vi "BPCS-Malicious-DE.vi"() -> ()   [LabVIEW 2017]
uses:
  <vilib>/Platform/TimedLoop/XDataNode/timing_clust.ctl
  <vilib>/Platform/TimedLoop/XDataNode/nitl_modes.ctl
  <vilib>/Platform/TimedLoop/XDataNode/wakeup.ctl
  <vilib>/addons/control/pid/pid.llb/PID Advanced (DBL).vi
  <vilib>/Platform/TimedLoop/XDataNode/XDataNode.xnode
  <vilib>/Platform/TimedLoop/XDataNode/XDNodeRunTimeDep.lvlib
  <vilib>/addons/control/pid/NI_PID_pid.lvlib
panel:
  in  "stop":bool
  out "data out":string
  in  "Stop":bool
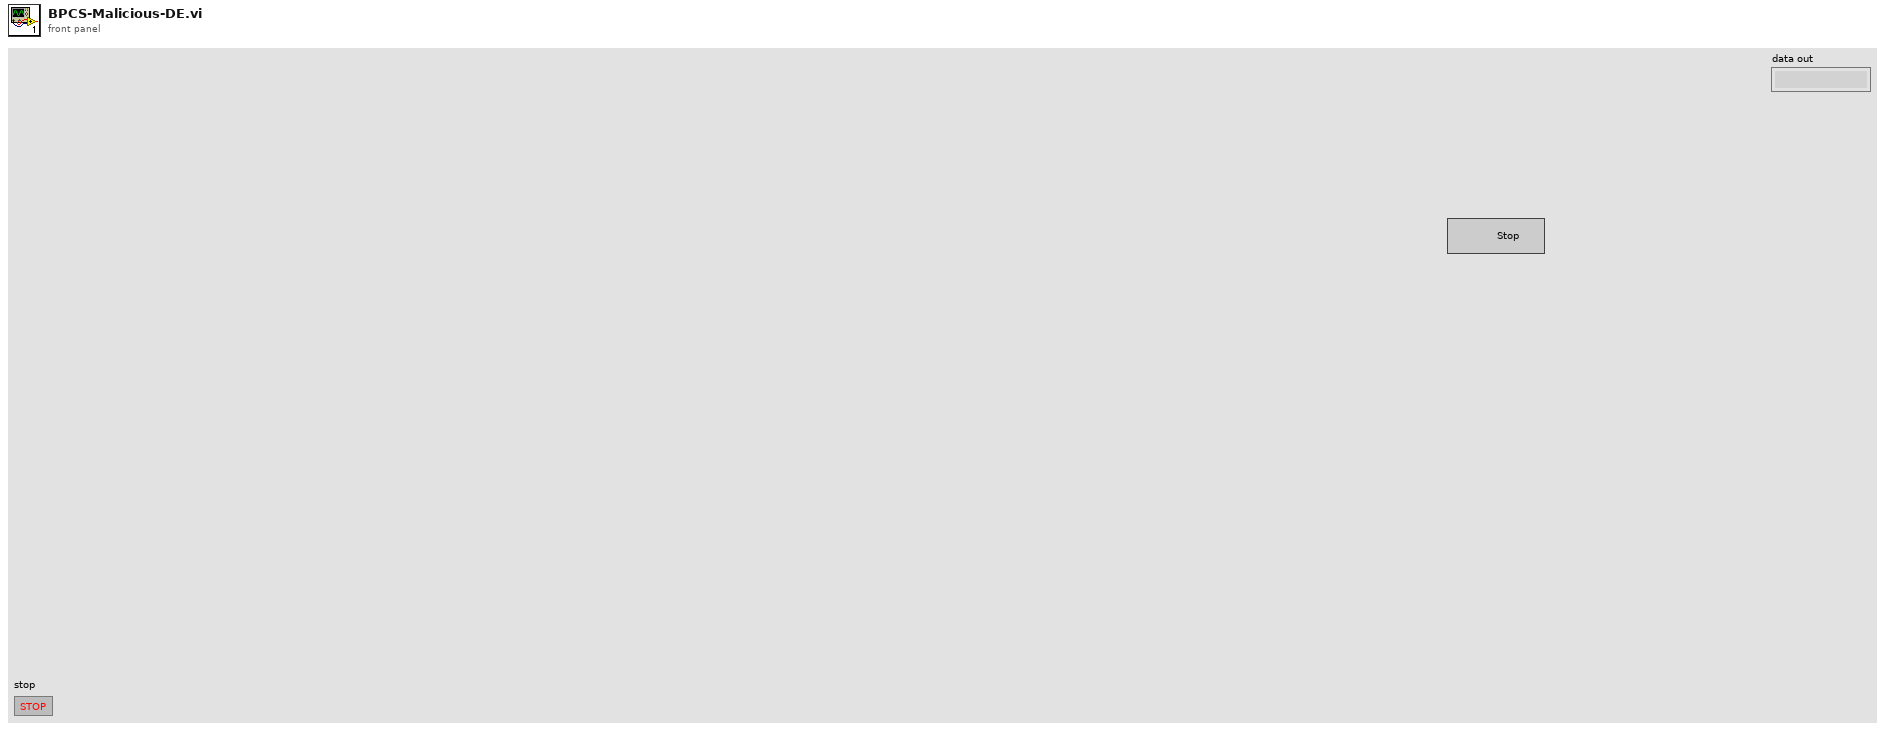
[diagram p1: front panel]
types:
  T1 = typedef "XDNodeRunTimeDep.lvlib/timing_clust.ctl" = cluster{"Expected End [f-1]":u64, "Actual End [f-1]":u64, "Finished Late? [f-1]":bool, "Expected End [i-1]":u64, "Actual End [i-1]":u64, "Finished Late? [i-1]":bool, "Expected Start [i]":u64, "Actual Start [i]":u64, "Expected Start [f]":u64, "Actual Start [f]":u64, "Source Name":string, "Structure Name":string, "Period":i64, "Deadline":i64, "Offset":i64, "Start":i64, "Priority":i32, "Timeout":i32, "Mode":T2, "Wakeup Reason":T3, "Error":errorcluster, "Source Type":string, "Secondary Source Type":string, "Global End Time":u64, "Global Start Time":u64, "Frame Duration":u64, "Iteration Duration":u64, "Assigned CPU":i32, "I/O Scan Engine Mode":u32}
  T2 = typedef "XDNodeRunTimeDep.lvlib/nitl_modes.ctl" = enum32{"No Change", "Process missed periods, maintain original phase", "Discard missed periods, maintain original phase", "Process missed periods, ignore original phase", "Discard missed periods, ignore original phase"}
  T3 = typedef "XDNodeRunTimeDep.lvlib/wakeup.ctl" = enum32{"Normal", "Aborted", "Asynchronous wakeup", "Timing source error", "Timed loop error", "Timeout"}
  T4 = cluster{"Array of Double[0]":dbl, "Array of Double[1]":dbl, "Array of Double[2]":dbl}
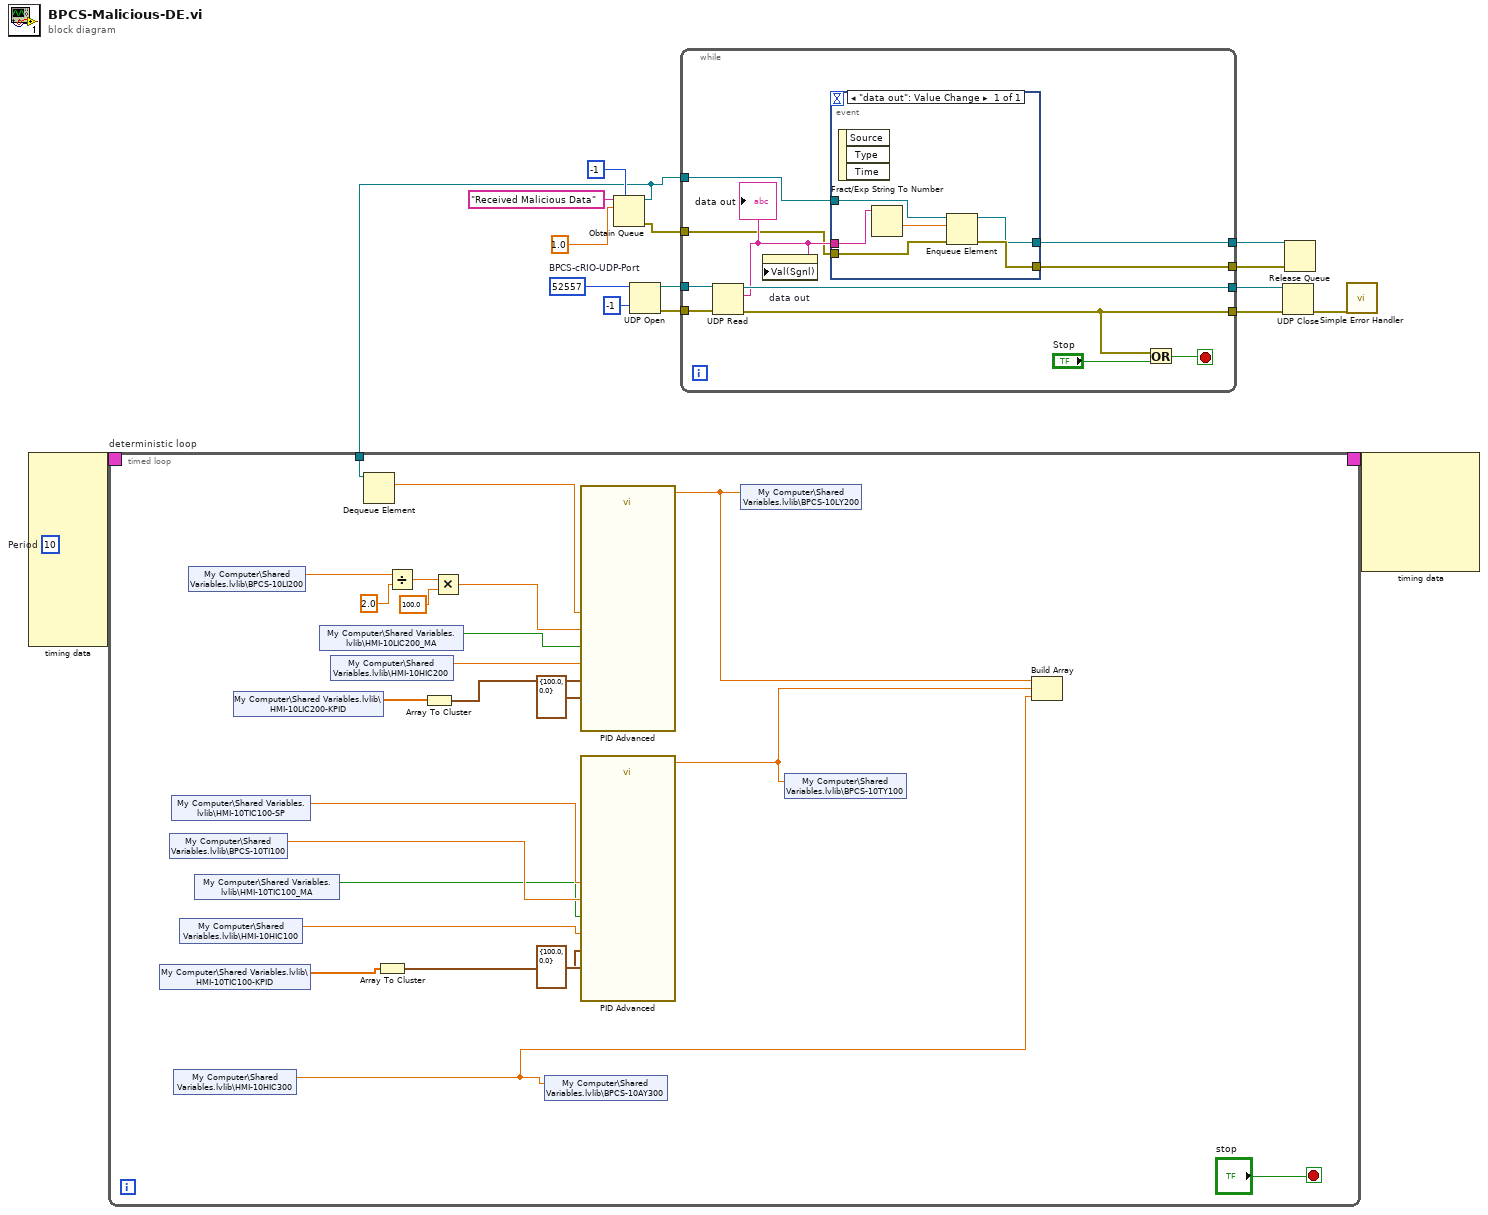
[diagram p0: block diagram]
diagram:
  w2 = i64 10  # Period
  w17 = u16 52557  # BPCS-cRIO-UDP-Port
  n1 = node-c288 ("Input Node")(w2) -> (w4:T1)  [unwired: 9 in]
  n2 = Obtain Queue(max queue size (-1, unlimited)=-1, name (unnamed)="Received Malicious Data", element data type=1.0) -> (queue out=w1:refnum<queue>, error out=w5:errorcluster)  [unwired: 2 in, 1 out]
  n3 = timed-loop "deterministic loop" {
    timing: w4 -> [_]
    timing-out: [_] -> w3
    tunnel: w1 -> [w19]
    stop <- "stop" stop-if-true
    n4 = shared-variable "My Computer\\Shared Variables.lvlib\\HMI-10TIC100-KPID"() -> (w25:dbl[])  [unwired: 1 in, 1 out]
    n5 = shared-variable "My Computer\\Shared Variables.lvlib\\BPCS-10TI100"() -> (w28:dbl)  [unwired: 1 in, 1 out]
    n6 = shared-variable "My Computer\\Shared Variables.lvlib\\HMI-10TIC100-SP"() -> (w29:dbl)  [unwired: 1 in, 1 out]
    n7 = shared-variable "My Computer\\Shared Variables.lvlib\\HMI-10HIC300"() -> (w20:dbl)  [unwired: 1 in, 1 out]
    n8 = shared-variable "My Computer\\Shared Variables.lvlib\\HMI-10HIC100"() -> (w26:dbl)  [unwired: 1 in, 1 out]
    n9 = shared-variable "My Computer\\Shared Variables.lvlib\\BPCS-10LI200"() -> (w37:dbl)  [unwired: 1 in, 1 out]
    n10 = shared-variable "My Computer\\Shared Variables.lvlib\\HMI-10TIC100_MA"() -> (w27:bool)  [unwired: 1 in, 1 out]
    n11 = shared-variable "My Computer\\Shared Variables.lvlib\\HMI-10LIC200-KPID"() -> (w36:dbl[])  [unwired: 1 in, 1 out]
    n12 = shared-variable "My Computer\\Shared Variables.lvlib\\HMI-10LIC200_MA"() -> (w32:bool)  [unwired: 1 in, 1 out]
    n13 = shared-variable "My Computer\\Shared Variables.lvlib\\HMI-10HIC200"() -> (w33:dbl)  [unwired: 1 in, 1 out]
    n14 = Dequeue Element(queue=w19) -> (element=w18:dbl)  [unwired: 2 in, 3 out]
    n15 = Array To Cluster(array=w25) -> (cluster=w24:T4)
    n16 = Divide(x=w37, y=2.0 ("x")) -> (x/y=w39:dbl)
    n17 = Array To Cluster(array=w36) -> (cluster=w34:T4)
    n18 = Multiply(x=w39, y=100.0) -> (x*y=w35:dbl)
    n19 = shared-variable "My Computer\\Shared Variables.lvlib\\BPCS-10AY300"(w20) -> ()  [unwired: 1 in, 1 out]
    n20 = call-poly <vilib>:"PID Advanced.vi"("setpoint"=w18, "output range"=cluster{"output high":dbl, "output low":dbl} {"output high"=100.0, "output low"=0.0}, "auto? (T)"=w32, "manual control"=w33, "process variable"=w35, "PID gains"=w34) -> ("output"=w22:dbl)  [unwired: 8 in, 1 out]
    n21 = call-poly <vilib>:"PID Advanced.vi"("setpoint"=w29, "output range"=cluster{"output high":dbl, "output low":dbl} {"output high"=100.0, "output low"=0.0}, "auto? (T)"=w27, "manual control"=w26, "process variable"=w28, "PID gains"=w24) -> ("output"=w21:dbl)  [unwired: 8 in, 1 out]
    n22 = shared-variable "My Computer\\Shared Variables.lvlib\\BPCS-10LY200"(w22) -> ()  [unwired: 1 in, 1 out]
    n23 = shared-variable "My Computer\\Shared Variables.lvlib\\BPCS-10TY100"(w21) -> ()  [unwired: 1 in, 1 out]
    n24 = Build Array(w22, w21, w20) -> ()  [unwired: 1 out]
  }
  n25 = UDP Open(9:-1 ("timeout ms (25000)"), 11:w17) -> (port=w16:refnum<k16>, 0:w15:errorcluster)  [unwired: 3 in, 1 out]
  n26 = while {
    tunnel: w16 -> [w51]
    tunnel: w15 -> [w50]
    tunnel: [w49] -> w13
    tunnel: [w48] -> w12
    tunnel: [w47] -> w7
    tunnel: [w46] -> w6
    tunnel: w1 -> [w44]
    tunnel: w5 -> [w43]
    stop <- w52 stop-if-true
    n27 = UDP Read(connection ID=w51, 8:w50) -> (data out=w45:string, error out=w48:errorcluster, 3:w49:refnum<k16>)  [unwired: 1 in, 3 out]
    "data out" <- w45
    n28 = property on="data out" class="Str"("Val(Sgnl)"=w45) -> ()  [unwired: 2 in, 2 out]
    n29 = event shown="[0] \"data out\": Value Change" {
      selector: _ -> [_]
      dyn-events: _ -> [_]
      timeout: _ -> [_]
      tunnel: [w58] -> w47
      tunnel: [w57] -> w46
      tunnel: w45 -> [w56]
      tunnel: w44 -> [w55]
      tunnel: w43 -> [w54]
      event "data out": Value Change {
        n30 = event-data() -> ()  [unwired: 1 in, 3 out]
        n31 = Fract/Exp String To Number(string=w56) -> (number=w59:dbl)  [unwired: 3 in, 1 out]
        n32 = Enqueue Element(queue=w55, element=w59, error in (no error)=w54) -> (queue out=w57:refnum<queue>, error out=w58:errorcluster)  [unwired: 1 in, 1 out]
      }
    }
    n33 = Or(x=w48, y="Stop") -> (x .or. y?=w52:bool)
  }
  n34 = UDP Close(connection ID=w13, 8:w12) -> (error out=w14:errorcluster)  [unwired: 1 out]
  n35 = Release Queue(queue=w6, error in (no error)=w7) -> ()  [unwired: 1 in, 3 out]
  n36 = call <vilib>:"Simple Error Handler.vi"("error in (no error)"=w14) -> ()  [unwired: 4 in, 5 out]
  n37 = node-c288 ("Output Node")(w3) -> ()  [unwired: 6 out]
